vi "Process Parameter Values.vi"(11 "Parameter Values":dbl[](array[numeric])) -> (3 "Processed Parameter Value Strings":string[](array[string]))   [LabVIEW 2020, in "Deep Reaction Optimizer Control Panel.lvlib" / "Logging.lvlib"]
uses:
  Logging.lvlib
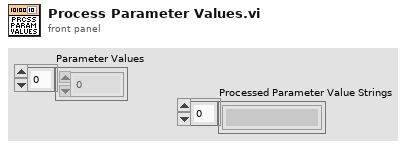
[diagram p1: front panel]
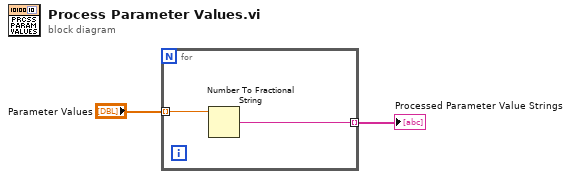
[diagram p0: block diagram]
diagram:
  n1 = for {
    tunnel: "Parameter Values" -> [w4] mode=indexing
    tunnel: [w3] -> w1 mode=indexing
    n2 = Number To Fractional String(number=w4) -> (F-format string=w3:string)  [unwired: 3 in]
  }
  "Processed Parameter Value Strings" <- w1
